vi "ARM Controller (SubVI).vi"(5 "alpha":i16 max=1023, 6 "Grip":i16 max=1023, 7 "J":i16 max=1023, 8 "error in (no error)":errorcluster, 9 "Z":i16 max=1023, 10 "R":i16 max=1023, 11 "teta":i16 max=1023) -> (0 "error out":errorcluster)   [LabVIEW 2017]
uses:
  <vilib>/myRIO/Instrument Drivers/Onboard IO/UART/typedef/VISA Configuration.ctl
  Projects/Auto control/Outputs.vi
  <vilib>/Instr/_visa.llb/VISA Configure Serial Port (Instr).vi
  <vilib>/myRIO/Express VI/Onboard IO/UART/UART Express VI.xnode
  <vilib>/myRIO/Instrument Drivers/Onboard IO/UART/UART.lvlib
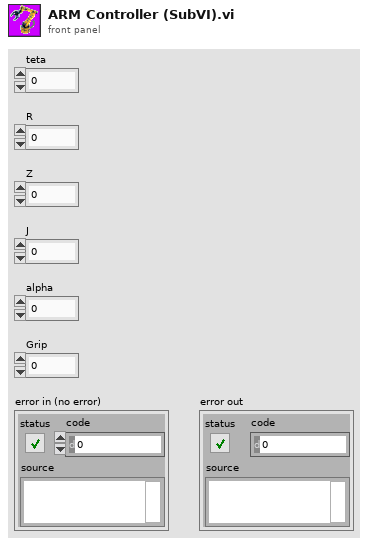
[diagram p1: front panel]
types:
  T1 = typedef "UART.lvlib/VISA Configuration.ctl" = cluster{"baud rate (9600)":u32, "data bits (8)":u16, "parity (0:none)":enum16{"None", "Odd", "Even", "Mark", "Space"}, "stop bits (10: 1 bit)":u16, "flow control (0:none)":u16, "termination char\n(0xA = '\\n' = LF) ":u8, "Enable Termination\nChar (T)":bool, "timeout (10sec)":u32}
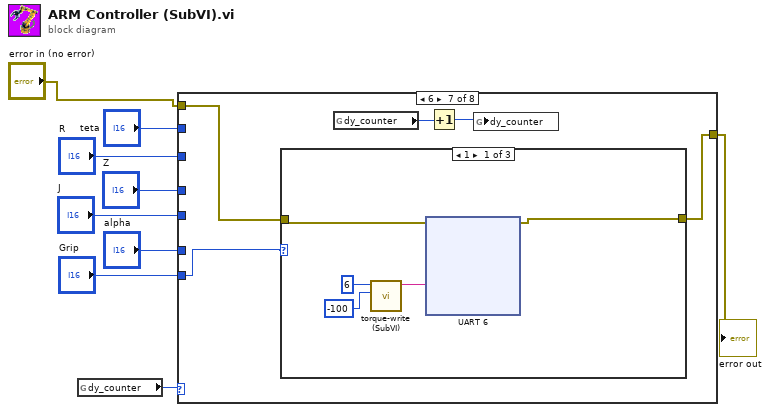
[diagram p0: block diagram]
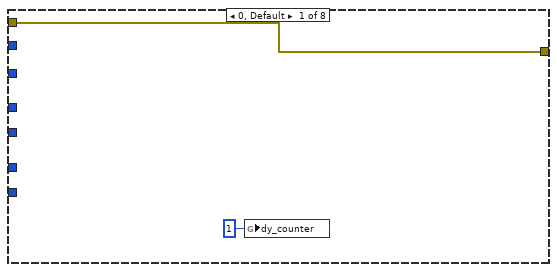
[diagram p2: hidden frame]
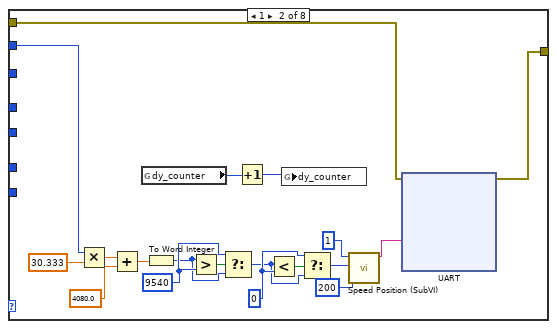
[diagram p3: hidden frame]
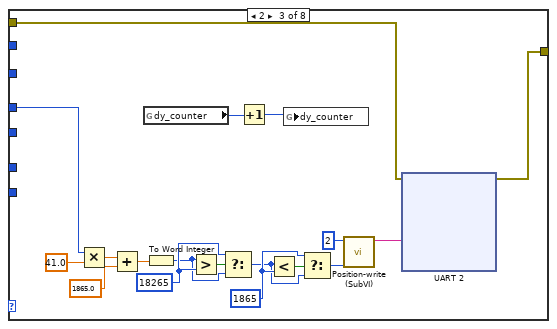
[diagram p4: hidden frame]
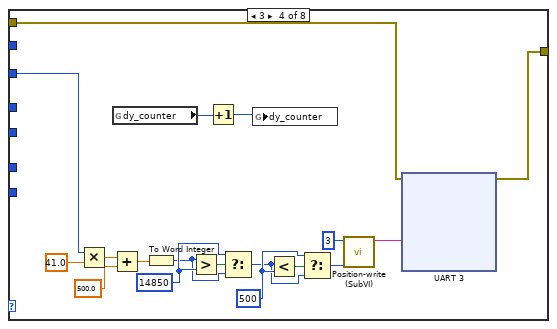
[diagram p5: hidden frame]
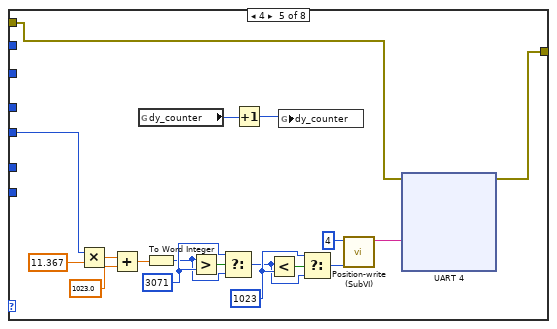
[diagram p6: hidden frame]
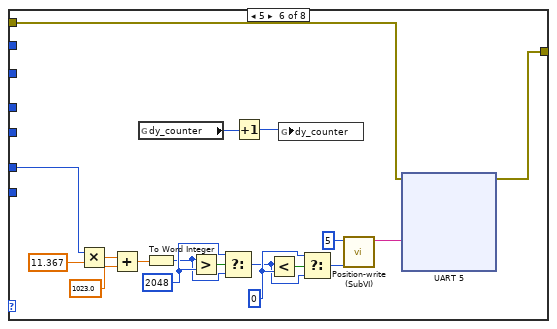
[diagram p7: hidden frame]
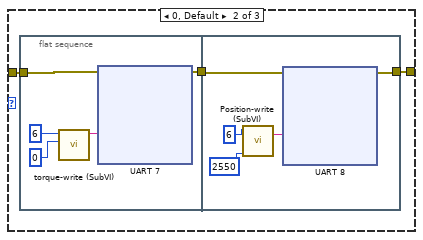
[diagram p8: hidden frame]
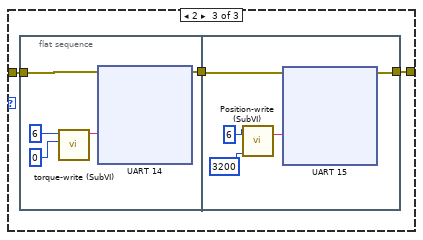
[diagram p9: hidden frame]
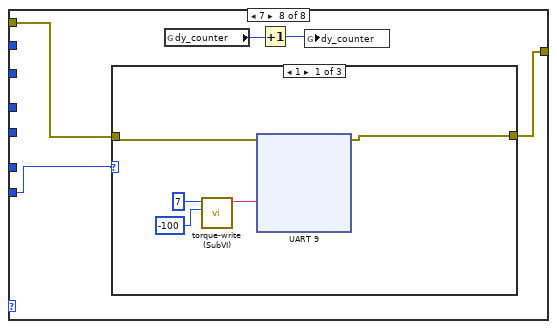
[diagram p10: hidden frame]
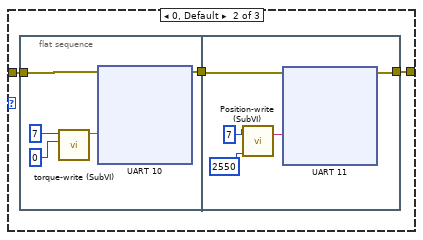
[diagram p11: hidden frame]
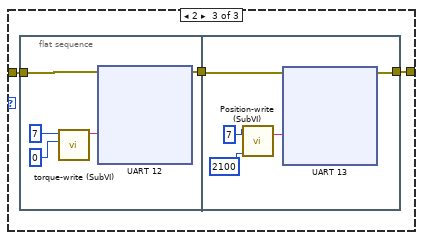
[diagram p12: hidden frame]
diagram:
  n1 = global read "Outputs.vi" "dy_counter"() -> (w7:i8)
  n2 = case shown="6" w7 {
    tunnel: "teta" -> [_ w20 _ _ _ _ _ _]
    tunnel: "R" -> [_ _ _ w85 _ _ _ _]
    tunnel: "Z" -> [_ _ w51 _ _ _ _ _]
    tunnel: "J" -> [_ _ _ _ w119 _ _ _]
    tunnel: "alpha" -> [_ _ _ _ _ w153 _ _]
    tunnel: "Grip" -> [_ _ _ _ _ _ w183 w299]
    tunnel: "error in (no error)" -> [w11 w19 w50 w84 w118 w152 w187 w303]
    tunnel: [w11 w18 w49 w83 w117 w151 w186 w302] -> w9
    frame 0, Default {
      n3 = global write "Outputs.vi" "dy_counter"(i8 1 ("dy_counter")) -> ()
    }
    frame 1 {
      w24 = i16 0 ("y")
      w26 = i16 9540 ("y")
      n4 = Multiply(x=w20, y=30.333) -> (x*y=w29:dbl)
      n5 = Add(x=w29, y=4080.0) -> (x+y=w22:dbl)
      n6 = global read "Outputs.vi" "dy_counter"() -> (w17:i8)
      n7 = To Word Integer(number=w22) -> (16bit integer=w21:i16)
      n8 = Greater?(x=w21, y=w26) -> (0:w27:bool)
      n9 = Select(t=w26, s=w27, f=w21) -> (s? t:f=w23:i16)
      n10 = Increment(x=w17) -> (x+1=w16:i8)
      n11 = Less?(x=w23, y=w24) -> (x < y?=w25:bool)
      n12 = global write "Outputs.vi" "dy_counter"(w16) -> ()
      n13 = Select(t=w24, s=w25, f=w23) -> (s? t:f=w13:i16)
      n14 = call "Speed Position (SubVI).vi"("Speed"=i16 200, "Position"=w13, "ID"=u8 1) -> ("result string"=w15:string)  [unwired: 8 in]
      n15 = xnode "UART"("Characters to Write"=w15, "error in (no error)"=w19) -> ("error out"=w18:errorcluster)  [unwired: 1 out]
    }
    frame 2 {
      w58 = i16 1865 ("y")
      w60 = i16 18265 ("y")
      n16 = Multiply(x=w51, y=41.0) -> (x*y=w63:dbl)
      n17 = Add(x=w63, y=1865.0) -> (x+y=w55:dbl)
      n18 = global read "Outputs.vi" "dy_counter"() -> (w48:i8)
      n19 = To Word Integer(number=w55) -> (16bit integer=w54:i16)
      n20 = Greater?(x=w54, y=w60) -> (0:w61:bool)
      n21 = Select(t=w60, s=w61, f=w54) -> (s? t:f=w57:i16)
      n22 = Increment(x=w48) -> (x+1=w47:i8)
      n23 = Less?(x=w57, y=w58) -> (x < y?=w59:bool)
      n24 = global write "Outputs.vi" "dy_counter"(w47) -> ()
      n25 = Select(t=w58, s=w59, f=w57) -> (s? t:f=w53:i16)
      n26 = call "Position-write (SubVI).vi"("Position"=w53, "ID"=u8 2) -> ("result string"=w56:string)  [unwired: 7 in]
      n27 = xnode "UART 2"("Characters to Write"=w56, "error in (no error)"=w50) -> ("error out"=w49:errorcluster)  [unwired: 1 out]
    }
    frame 3 {
      w92 = i16 500 ("y")
      w94 = i16 14850 ("y")
      n28 = Multiply(x=w85, y=41.0) -> (x*y=w97:dbl)
      n29 = Add(x=w97, y=500.0) -> (x+y=w89:dbl)
      n30 = global read "Outputs.vi" "dy_counter"() -> (w82:i8)
      n31 = To Word Integer(number=w89) -> (16bit integer=w88:i16)
      n32 = Greater?(x=w88, y=w94) -> (0:w95:bool)
      n33 = Increment(x=w82) -> (x+1=w81:i8)
      n34 = Select(t=w94, s=w95, f=w88) -> (s? t:f=w91:i16)
      n35 = global write "Outputs.vi" "dy_counter"(w81) -> ()
      n36 = Less?(x=w91, y=w92) -> (x < y?=w93:bool)
      n37 = Select(t=w92, s=w93, f=w91) -> (s? t:f=w87:i16)
      n38 = call "Position-write (SubVI).vi"("Position"=w87, "ID"=u8 3) -> ("result string"=w90:string)  [unwired: 7 in]
      n39 = xnode "UART 3"("Characters to Write"=w90, "error in (no error)"=w84) -> ("error out"=w83:errorcluster)  [unwired: 1 out]
    }
    frame 4 {
      w126 = i16 1023 ("y")
      w128 = i16 3071 ("y")
      n40 = Multiply(x=w119, y=11.367) -> (x*y=w131:dbl)
      n41 = Add(x=w131, y=1023.0) -> (x+y=w123:dbl)
      n42 = global read "Outputs.vi" "dy_counter"() -> (w116:i8)
      n43 = To Word Integer(number=w123) -> (16bit integer=w122:i16)
      n44 = Greater?(x=w122, y=w128) -> (0:w129:bool)
      n45 = Select(t=w128, s=w129, f=w122) -> (s? t:f=w125:i16)
      n46 = Increment(x=w116) -> (x+1=w115:i8)
      n47 = Less?(x=w125, y=w126) -> (x < y?=w127:bool)
      n48 = global write "Outputs.vi" "dy_counter"(w115) -> ()
      n49 = Select(t=w126, s=w127, f=w125) -> (s? t:f=w121:i16)
      n50 = call "Position-write (SubVI).vi"("Position"=w121, "ID"=u8 4) -> ("result string"=w124:string)  [unwired: 7 in]
      n51 = xnode "UART 4"("Characters to Write"=w124, "error in (no error)"=w118) -> ("error out"=w117:errorcluster)  [unwired: 1 out]
    }
    frame 5 {
      w160 = i16 0 ("y")
      w162 = i16 2048 ("y")
      n52 = Multiply(x=w153, y=11.367) -> (x*y=w165:dbl)
      n53 = Add(x=w165, y=1023.0) -> (x+y=w157:dbl)
      n54 = global read "Outputs.vi" "dy_counter"() -> (w150:i8)
      n55 = To Word Integer(number=w157) -> (16bit integer=w156:i16)
      n56 = Greater?(x=w156, y=w162) -> (0:w163:bool)
      n57 = Select(t=w162, s=w163, f=w156) -> (s? t:f=w159:i16)
      n58 = Increment(x=w150) -> (x+1=w149:i8)
      n59 = Less?(x=w159, y=w160) -> (x < y?=w161:bool)
      n60 = global write "Outputs.vi" "dy_counter"(w149) -> ()
      n61 = Select(t=w160, s=w161, f=w159) -> (s? t:f=w155:i16)
      n62 = call "Position-write (SubVI).vi"("Position"=w155, "ID"=u8 5) -> ("result string"=w158:string)  [unwired: 7 in]
      n63 = xnode "UART 5"("Characters to Write"=w158, "error in (no error)"=w152) -> ("error out"=w151:errorcluster)  [unwired: 1 out]
    }
    frame 6 {
      n64 = case shown="1" w183 {
        tunnel: w187 -> [w192 w211 w256]
        tunnel: [w188 w210 w255] -> w186
        frame 1 {
          n65 = call "torque-write (SubVI).vi"("Torque"=i16 -100 ("Position"), "ID"=u8 6) -> ("result string"=w190:string)  [unwired: 9 in]
          n66 = xnode "UART 6"("Characters to Write"=w190, "error in (no error)"=w192) -> ("error out"=w188:errorcluster)  [unwired: 1 out]
        }
        frame 0, Default {
          n67 = flat-sequence {
            tunnel: w211 -> [w216]
            tunnel: [w212] -> w209
            tunnel: [w236] -> w210
            tunnel: w209 -> [w237]
            frame #0 {
              n68 = call "torque-write (SubVI).vi"("Torque"=i16 0 ("Position"), "ID"=u8 6) -> ("result string"=w214:string)  [unwired: 9 in]
              n69 = xnode "UART 7"("Characters to Write"=w214, "error in (no error)"=w216) -> ("error out"=w212:errorcluster)  [unwired: 1 out]
            }
            frame #1 {
              n70 = call "Position-write (SubVI).vi"("Position"=i16 2550, "ID"=u8 6) -> ("result string"=w234:string)  [unwired: 7 in]
              n71 = xnode "UART 8"("Characters to Write"=w234, "error in (no error)"=w237) -> ("error out"=w236:errorcluster)  [unwired: 1 out]
            }
          }
        }
        frame 2 {
          n72 = flat-sequence {
            tunnel: w256 -> [w261]
            tunnel: [w257] -> w254
            tunnel: [w281] -> w255
            tunnel: w254 -> [w282]
            frame #0 {
              n73 = call "torque-write (SubVI).vi"("Torque"=i16 0 ("Position"), "ID"=u8 6) -> ("result string"=w259:string)  [unwired: 9 in]
              n74 = xnode "UART 14"("Characters to Write"=w259, "error in (no error)"=w261) -> ("error out"=w257:errorcluster)  [unwired: 1 out]
            }
            frame #1 {
              n75 = call "Position-write (SubVI).vi"("Position"=i16 3200, "ID"=u8 6) -> ("result string"=w279:string)  [unwired: 7 in]
              n76 = xnode "UART 15"("Characters to Write"=w279, "error in (no error)"=w282) -> ("error out"=w281:errorcluster)  [unwired: 1 out]
            }
          }
        }
      }
      n77 = global read "Outputs.vi" "dy_counter"() -> (w185:i8)
      n78 = Increment(x=w185) -> (x+1=w184:i8)
      n79 = global write "Outputs.vi" "dy_counter"(w184) -> ()
    }
    frame 7 {
      n80 = case shown="1" w299 {
        tunnel: w303 -> [w308 w327 w372]
        tunnel: [w304 w326 w371] -> w302
        frame 1 {
          n81 = call "torque-write (SubVI).vi"("Torque"=i16 -100 ("Position"), "ID"=u8 7) -> ("result string"=w306:string)  [unwired: 9 in]
          n82 = xnode "UART 9"("Characters to Write"=w306, "error in (no error)"=w308) -> ("error out"=w304:errorcluster)  [unwired: 1 out]
        }
        frame 0, Default {
          n83 = flat-sequence {
            tunnel: w327 -> [w332]
            tunnel: [w328] -> w325
            tunnel: [w352] -> w326
            tunnel: w325 -> [w353]
            frame #0 {
              n84 = call "torque-write (SubVI).vi"("Torque"=i16 0 ("Position"), "ID"=u8 7) -> ("result string"=w330:string)  [unwired: 9 in]
              n85 = xnode "UART 10"("Characters to Write"=w330, "error in (no error)"=w332) -> ("error out"=w328:errorcluster)  [unwired: 1 out]
            }
            frame #1 {
              n86 = call "Position-write (SubVI).vi"("Position"=i16 2550, "ID"=u8 7) -> ("result string"=w350:string)  [unwired: 7 in]
              n87 = xnode "UART 11"("Characters to Write"=w350, "error in (no error)"=w353) -> ("error out"=w352:errorcluster)  [unwired: 1 out]
            }
          }
        }
        frame 2 {
          n88 = flat-sequence {
            tunnel: w372 -> [w377]
            tunnel: [w373] -> w370
            tunnel: [w397] -> w371
            tunnel: w370 -> [w398]
            frame #0 {
              n89 = call "torque-write (SubVI).vi"("Torque"=i16 0 ("Position"), "ID"=u8 7) -> ("result string"=w375:string)  [unwired: 9 in]
              n90 = xnode "UART 12"("Characters to Write"=w375, "error in (no error)"=w377) -> ("error out"=w373:errorcluster)  [unwired: 1 out]
            }
            frame #1 {
              n91 = call "Position-write (SubVI).vi"("Position"=i16 2100, "ID"=u8 7) -> ("result string"=w395:string)  [unwired: 7 in]
              n92 = xnode "UART 13"("Characters to Write"=w395, "error in (no error)"=w398) -> ("error out"=w397:errorcluster)  [unwired: 1 out]
            }
          }
        }
      }
      n93 = global read "Outputs.vi" "dy_counter"() -> (w301:i8)
      n94 = Increment(x=w301) -> (x+1=w300:i8)
      n95 = global write "Outputs.vi" "dy_counter"(w300) -> ()
    }
  }
  "error out" <- w9
